vi "startUp.vi"(8 "error in (no error)":errorcluster, 10 "HardwareList out":refnum<class "HWConfiguration.lvclass">, 11 "HWController in":refnum<class "HWController.lvclass">) -> (0 "error out":errorcluster, 3 "HWController out":refnum<class "HWController.lvclass">)   [LabVIEW 2011, in "Hardware.lvlib" / "HWControllers.lvlib" / "HWController.lvclass"]
doc: "Startsup the hardware controller"
uses:
  HWController.lvclass
  HardwareConfiguration/HWConfiguration.lvclass
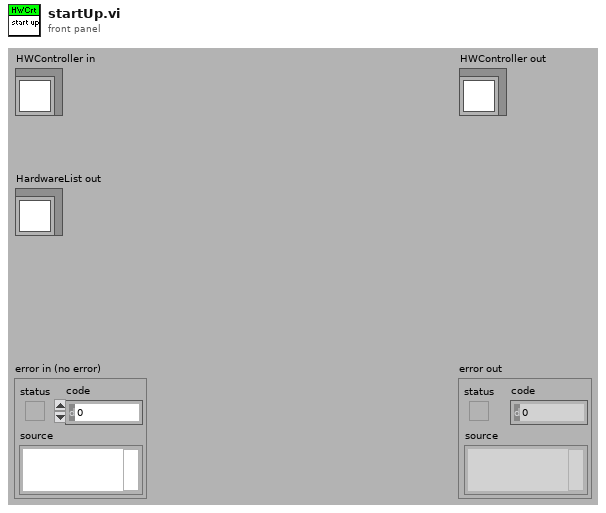
[diagram p1: front panel]
types:
  T1 = enum16{"Ready", "Compiling", "Configured", "Running", "Stopping", "Unresolved Error"}
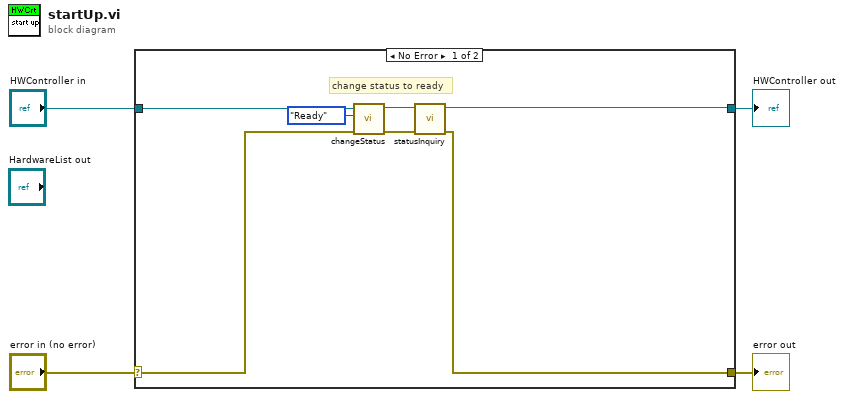
[diagram p0: block diagram]
diagram:
  n1 = case shown="No Error" "error in (no error)" {
    selector: "error in (no error)" -> [w7 w13]
    tunnel: [w6 w13] -> w3
    tunnel: [w8 w12] -> w1
    tunnel: "HWController in" -> [w9 w12]
    frame No Error {
      # "change status to ready"
      n2 = call "changeStatus.vi"("error in (no error)"=w7, "status"=T1."Ready", "HWController in"=w9) -> ("error out"=w11:errorcluster, "HWController out"=w10:refnum<class "HWController.lvclass">)  [unwired: 7 in]
      n3 = call-dynamic "statusInquiry.vi"("error in (no error)"=w11, "HWController in"=w10) -> ("error out"=w6:errorcluster, "HWController out"=w8:refnum<class "HWController.lvclass">)  [unwired: 8 in]
    }
    frame Error {
    }
  }
  "error out" <- w3
  "HWController out" <- w1
